vi "2_VisualAD__Inference(Image).vi"() -> ()   [LabVIEW 2020]
uses:
  <vilib>/Ngene/DeepLTK Anomaly Detection Addon/DeepLTK_Anomaly_Detection_Addon/API/Controls/NNPC_Setup.ctl
  <vilib>/Ngene/Deep Learning Toolkit/Toolkit/NN_Data/API/NN_Dims(C,H,W).ctl
  <vilib>/Ngene/Deep Learning Toolkit/Toolkit/NN_Network/Controls/NN_Device.ctl
  <vilib>/Ngene/DeepLTK Anomaly Detection Addon/DeepLTK_Anomaly_Detection_Addon/API/Controls/Feature_Scorer_Params.ctl
  <vilib>/Ngene/DeepLTK Anomaly Detection Addon/DeepLTK_Anomaly_Detection_Addon/API/Controls/Gaussian_Blur.ctl
  <vilib>/Ngene/DeepLTK Anomaly Detection Addon/DeepLTK_Anomaly_Detection_Addon/API/Controls/NN_Paths.ctl
  subVIs/Visualizer/Controls/Display_Options.ctl
  subVIs/Visualizer/Controls/ROI_Display_Options.ctl
  subVIs/Visualizer/Controls/Heatmap_Display_Options.ctl
  subVIs/Visualizer/Controls/ColorMap.ctl
  <vilib>/Ngene/DeepLTK Anomaly Detection Addon/DeepLTK_Anomaly_Detection_Addon/API/Controls/MinMax.ctl
  <vilib>/Ngene/DeepLTK Anomaly Detection Addon/DeepLTK_Anomaly_Detection_Addon/API/NNPC_Predict/NNPC_Predict(Single).vi
  <vilib>/ptbypt/NI_PtbyPt.lvlib
  <vilib>/Ngene/DeepLTK Anomaly Detection Addon/DeepLTK_Anomaly_Detection_Addon/DeepLTK_Anomaly_Detection_Addon.lvlib
  <vilib>/Ngene/Deep Learning Toolkit/Toolkit/Deep_Learning_Toolkit_by_Ngene.lvlib
panel:
  in  "Display_Options":T1={"ROI_Options"={"Color"=16383, "Width"=3, "Drawing Mode"=enum."Frame"}, "Heatmap_Options"={"ColorMap"=enum."Jet", "Alpha"=0.4, "Heatmap_Range"={"Min"=-1.0, "Max"=-1.0}}, "Has GT?"=FALSE} {"Heatmap_Options"."Heatmap_Range"."Min" format="%#_5g"}
  out "dT_Init":dbl=3.8699048000016774 format="%#_3ps"
  in  "NNPC_Paths":T6={"CFG"=path "D:/Ngene/GitHub/deepltk_examples/3_Image_Processing/36_Anomaly_Detection/Models/NNPC_Cards_3ofHearts__25_03_28__20_34_36/NNPC_Cards_3ofHearts.cfg", "BIN"=path "D:/Ngene/GitHub/deepltk_examples/3_Image_Processing/36_Anomaly_Detection/Models/NNPC_Cards_3ofHearts__25_03_28__20_34_36/NNPC_Cards_3ofHearts.bin"}
  out "Image_Thrshld (Eval)":sgl=11.161
  in  "Image_Thrshld(Custom)":sgl=-1.0 format="%_5g"
  out "dT_Predict":dbl=0.005395784000138519 format="%#_3ps"
  out "Pixel_Score(Min)":sgl=1.6810824
  out "Pixel_Score(Max)":sgl=12.34793
  out "Image_File_Path":path=path "D:/Ngene/GitHub/deepltk_examples/3_Image_Processing/36_Anomaly_Detection/Dataset/Playing_Cards_3ofHearts/test/bad/(159).png"
  in  "Feature_Scorer_Params":T7={"Nearest_Neighbors"=1, "Calculate Anomaly Map"=TRUE, "Gaussian_Blur"={"Kernel_Size"=33, "Sigma"=4.0}}
  out "Pixel_Thrshld (Eval)":sgl=2.5442
  in  "Stop":bool
  out "Anomaly?":bool=TRUE
  out "dT_ImRead":dbl=0.002829499997460516 format="%#_4ps"
  in  "NNPC_Setup":T9={"Input_Dims"={"C"=-1, "H"=-1, "W"=-1}, "mBatch"=1, "Device"=enum."GPU", "GPU Id"=0}
  out "Anomaly Detection Results":T12(plugin-control)
  out "Img_Score":sgl=14.09682
  in  "Image_idx":u32=33 max=49
  in  "Ground_Truth_Folder_Path":path
  in  "Pixel_Thrshld(Custom)":sgl=10.0 format="%_5g"
  in  "Test_Dataset_Folder_Path":path=path "D:/Ngene/GitHub/deepltk_examples/3_Image_Processing/36_Anomaly_Detection/Dataset/Playing_Cards_3ofHearts/test"
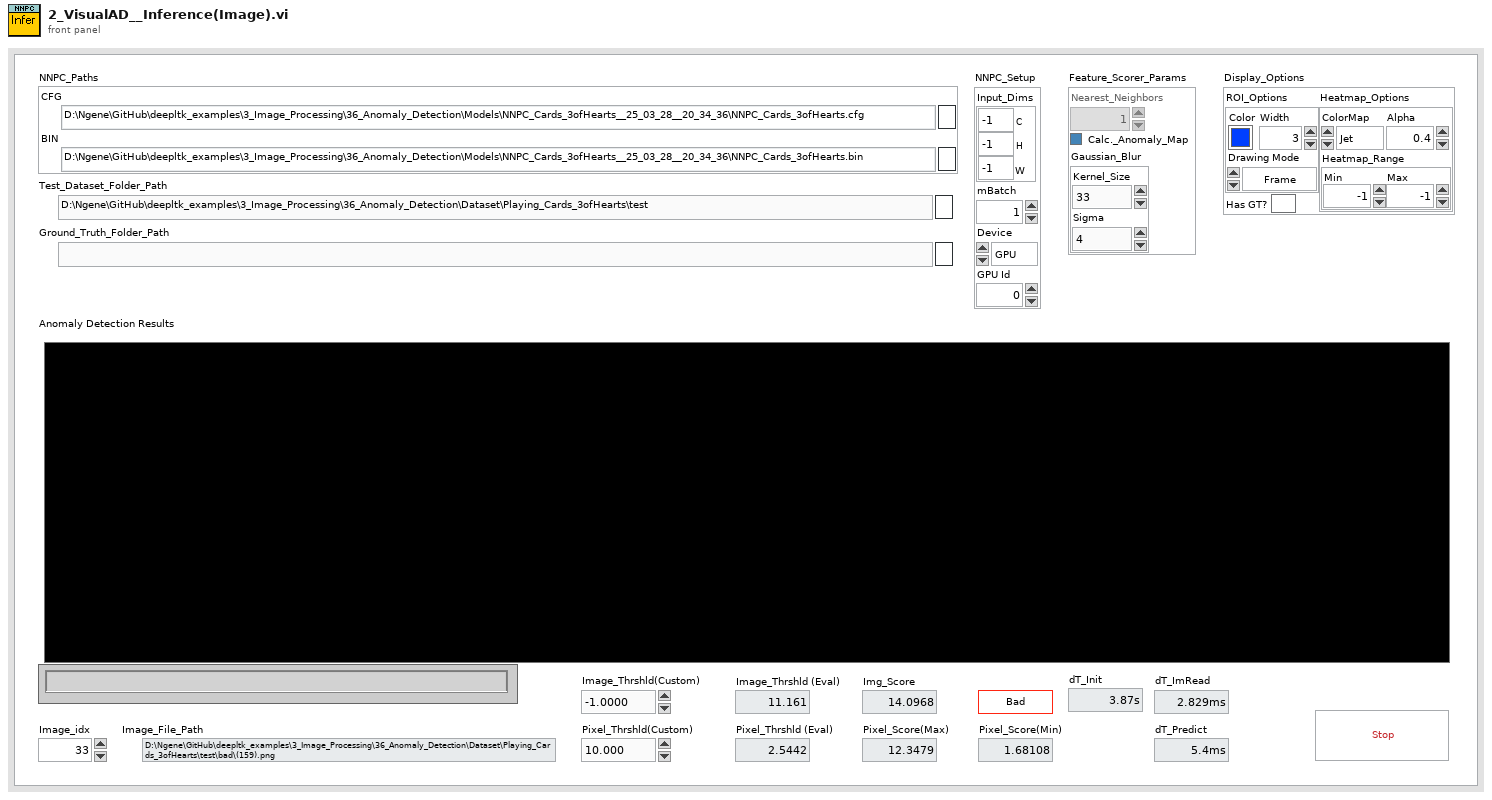
[diagram p1: front panel]
types:
  T1 = typedef "Display_Options.ctl" = cluster{"ROI_Options":T2, "Heatmap_Options":T3, "Has GT?":bool}
  T2 = typedef "ROI_Display_Options.ctl" = cluster{"Color":u32, "Width":u32, "Drawing Mode":enum16{"Frame", "Fill"}}
  T3 = typedef "Heatmap_Display_Options.ctl" = cluster{"ColorMap":T4, "Alpha":sgl, "Heatmap_Range":T5}
  T4 = typedef "ColorMap.ctl" = enum16{"Jet", "Perula", "Inferno", "Plasma", "Viridis"}
  T5 = typedef "DeepLTK_Anomaly_Detection_Addon.lvlib/MinMax.ctl" = cluster{"Min":sgl, "Max":sgl}
  T6 = typedef "DeepLTK_Anomaly_Detection_Addon.lvlib/NN_Paths.ctl" = cluster{"CFG":path, "BIN":path}
  T7 = typedef "DeepLTK_Anomaly_Detection_Addon.lvlib/Feature_Scorer_Params.ctl" = cluster{"Nearest_Neighbors":i32, "Calculate Anomaly Map":bool, "Gaussian_Blur":T8}
  T8 = typedef "DeepLTK_Anomaly_Detection_Addon.lvlib/Gaussian_Blur.ctl" = cluster{"Kernel_Size":i32, "Sigma":sgl}
  T9 = typedef "DeepLTK_Anomaly_Detection_Addon.lvlib/NNPC_Setup.ctl" = cluster{"Input_Dims":T10, "mBatch":i32, "Device":T11, "GPU Id":i32}
  T10 = typedef "Deep_Learning_Toolkit_by_Ngene.lvlib/NN_Dims(C,H,W).ctl" = cluster{"C":i32, "H":i32, "W":i32}
  T11 = typedef "Deep_Learning_Toolkit_by_Ngene.lvlib/NN_Device.ctl" = enum16{"CPU", "GPU"}
  T12 = typedef "IMAQ Image.ctl" = refnum<image>
  T13 = typedef "DeepLTK_Anomaly_Detection_Addon.lvlib/NNPC_Evaluation_Results.ctl" = cluster{"Threshold(Image)":sgl, "Threshold(Pixel)":sgl, "Pixel_Range":cluster{"Min":sgl, "Max":sgl}}
  T14 = typedef "DeepLTK_Anomaly_Detection_Addon.lvlib/NNPC_PreProcessing_Options.ctl" = cluster{"DS_Name":string, "Input_Dims":T10, "Center Crop Size":i32, "Interpolation Type":u32, "Dataset_Stats":T15}
  T15 = typedef "DeepLTK_Anomaly_Detection_Addon.lvlib/NNPC_DS_Stats.ctl" = cluster{"means":T16, "stds":T16}
  T16 = typedef "DeepLTK_Anomaly_Detection_Addon.lvlib/Image_Stats_RGB.ctl" = cluster{"R":sgl, "G":sgl, "B":sgl}
  T17 = typedef "DeepLTK_Anomaly_Detection_Addon.lvlib/NNPC_Instance.ctl" = cluster{"NN":T18, "MemBank_Data":T33, "Name":string}
  T18 = typedef "Deep_Learning_Toolkit_by_Ngene.lvlib/NN.ctl" = cluster{"Name":string, "No of Layers":i32, "mBatch":i32, "Layers":T19[], "Dimty":T20, "Dims_In":T10, "Dims_Out":T10, "Working_Dir":path, "Train?":bool, "Train_Params":T21, "LR_Update_Policy":T24, "Session Data":T26, "Ground_truth":T27, "NNg_hdls":T28, "NN_Device":T11, "GPU Id":i32, "Labels":string[], "Receptive Field":T29[], "Loss_Type":T30, "Loss_Cfg_Prms":variant, "NNG_WS":T31}
  T19 = typedef "Deep_Learning_Toolkit_by_Ngene.lvlib/NN_Layer_ref.ctl" = refnum<data-value>
  T20 = typedef "Deep_Learning_Toolkit_by_Ngene.lvlib/NN_In_Out_Dim-ty.ctl" = enum8{"In1D_Out1D", "In3D_Out1D", "In3D_Out3D", "In3D_OutBBox"}
  T21 = typedef "Deep_Learning_Toolkit_by_Ngene.lvlib/NN_Train_Params.ctl" = cluster{"Optimizer":T22, "Beta_1":sgl, "Beta_2":sgl, "Weight Decay(L1)":sgl, "Weight Decay(L2)":sgl, "Data_Sampling":T23}
  T22 = typedef "Deep_Learning_Toolkit_by_Ngene.lvlib/NN_Train_Optimizer.ctl" = enum16{"SGD", "Adam", "Adagrad", "Adadelta", "RMSProp", "Nesterov"}
  T23 = typedef "Deep_Learning_Toolkit_by_Ngene.lvlib/NN_Train_Data_Sampling.ctl" = enum16{"Random", "Sequential"}
  T24 = typedef "Deep_Learning_Toolkit_by_Ngene.lvlib/NN_LR_Policy_Cfg.ctl" = cluster{"Policy_Type":T25, "LR0":dbl, "k":sgl, "WarmUp_Policy":enum16{"Step", "Ramp"}, "WarmUp_Iter":i32, "WarmUp_Ratio":sgl}
  T25 = typedef "Deep_Learning_Toolkit_by_Ngene.lvlib/NN_LR_Policy_Type.ctl" = enum16{"Manual", "Step", "Exp", "1/t"}
  T26 = typedef "Deep_Learning_Toolkit_by_Ngene.lvlib/NN_Train_Session_Data.ctl" = cluster{"Epochs":sgl, "Tot_Iter":i32, "LR":sgl, "LR_iter":i32}
  T27 = typedef "Deep_Learning_Toolkit_by_Ngene.lvlib/NN_Ground_truth.ctl" = cluster{"Y":variant}
  T28 = typedef "Deep_Learning_Toolkit_by_Ngene.lvlib/nng_cuda_handles.ctl" = cluster{"cudnn":u64, "cublas":u64, "stream":u64, "curand":u64}
  T29 = typedef "Deep_Learning_Toolkit_by_Ngene.lvlib/NN_Dims(V,H).ctl" = cluster{"V":i32, "H":i32}
  T30 = typedef "Deep_Learning_Toolkit_by_Ngene.lvlib/NN_Loss_Type.ctl" = enum16{"None", "MSE", "CrossEntropy", "YOLO_v2", "YOLO_v4"}
  T31 = typedef "Deep_Learning_Toolkit_by_Ngene.lvlib/NNG_WS.ctl" = cluster{"NNG_WS_Mem":T32, "Max_WS_Size":i64}
  T32 = typedef "Deep_Learning_Toolkit_by_Ngene.lvlib/NNg_WS_Mem_DVR.ctl" = refnum<data-value>
  T33 = typedef "DeepLTK_Anomaly_Detection_Addon.lvlib/MemBank_and_Norm_Variants.ctl" = cluster{"MemBank":variant, "MemBank Norm":variant}
  T34 = typedef "Anomaly_Detection_Results_Imgs.ctl" = cluster{"Image":T12, "Ground Truth":T12, "Predicted Heat Map":T12, "Predicted Mask":T12, "Segmentation":T12}
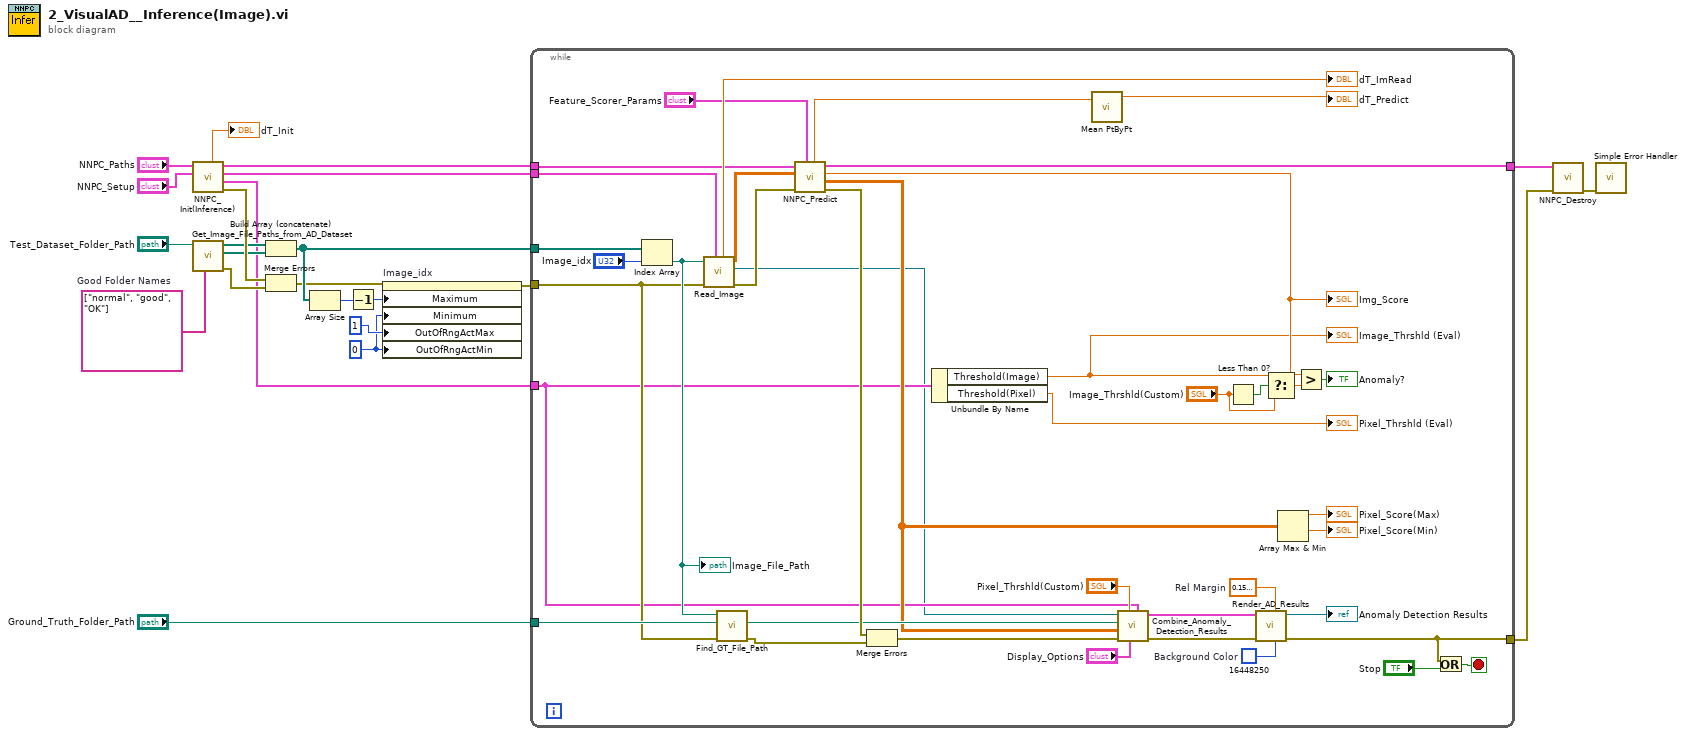
[diagram p0: block diagram]
diagram:
  w1 = string[] ["normal", "good", "OK"]  # Good Folder Names
  w3 = u32 0 ("Data Entry Limits:Minimum")
  n1 = call <vilib>:"NNPC_Init(Inference).vi"("NNPC_Setup"="NNPC_Setup", "NNPC_Paths"="NNPC_Paths") -> ("error out"=w21:errorcluster, "Evaluation_Results"=w4:T13, "PreProc_Options"=w6:T14, "NNPC_out"=w22:T17, "dT_Init_Inference"=→"dT_Init":dbl)  [unwired: 5 in]
  n2 = call "Get_Image_File_Paths_from_AD_Dataset.vi"("Good Folder Names"=w1, "Dataset Folder"="Test_Dataset_Folder_Path") -> ("error out"=w18:errorcluster, "Bad Dataset Files"=w14:path[], "Good Dataset Files"=w13:path[])  [unwired: 7 in]
  n3 = Build Array (concatenate)(w13, w14) -> (w19:path[])
  n4 = Merge Errors(w21, w18) -> (w8:errorcluster)
  n5 = Array Size(array=w19) -> (size(s)=w9:i32)
  n6 = Decrement(x=w9) -> (x-1=w11:i32)
  n7 = property on="Image_idx" class="DigNum (strict)"(error in=w8, "Maximum"=w11, "Minimum"=w3, "OutOfRngActMax"=u8 1 ("Response to Value Outside Limits:Maximum"), "OutOfRngActMin"=w3) -> (error out=w7:errorcluster)  [unwired: 1 in, 1 out]
  n8 = while {
    tunnel: w19 -> [w63]
    tunnel: w22 -> [w45]
    tunnel: [w39] -> w16
    tunnel: w7 -> [w34]
    tunnel: [w36] -> w17
    tunnel: "Ground_Truth_Folder_Path" -> [w48]
    tunnel: w6 -> [w31]
    tunnel: w4 -> [w27]
    stop <- w37 stop-if-true
    w35 = u32 16448250  # Background Color
    w55 = sgl 0.15  # Rel Margin
    n9 = Index Array(array=w63, index="Image_idx") -> (element=w50:path)
    "Image_File_Path" <- w50
    n10 = call "Read_Image.vi"("PreProcessing_Options"=w31, "error in"=w34, "Img Path"=w50) -> ("error out"=w40:errorcluster, "Imaq Image Out"=w26:T12, "Image Out"=w24:sgl[][][], "dT_Img_Read"=→"dT_ImRead":dbl)  [unwired: 5 in]
    n11 = call "Find_GT_File_Path.vi"("error in"=w34, "GT Mask Folder Path"=w48, "Image File Path"=w50) -> ("error out"=w32:errorcluster, "GT File Path"=w49:path)  [unwired: 5 in, 2 out]
    n12 = call-poly <vilib>:"NNPC_Predict.vi"("Feature_Scorer_Params"="Feature_Scorer_Params", "error in"=w40, "Image_in"=w24, "NNPC_in"=w45) -> ("error out"=w61:errorcluster, "Anomaly_Map"=w44:sgl[][], "Pred_Score"=w43:sgl, "NNPC_out"=w39:T17, "dT_Predict"=w30:dbl)  [unwired: 3 in]
    "Img_Score" <- w43
    n13 = Merge Errors(w61, w32) -> (w33:errorcluster)
    n14 = Unbundle By Name(w27) -> ("Threshold(Image)"=w29:sgl, "Threshold(Pixel)"=→"Pixel_Thrshld (Eval)":sgl)
    "Image_Thrshld (Eval)" <- w29
    n15 = call <vilib>:"Mean PtByPt.vi"("x"=w30) -> ("mean"=→"dT_Predict":dbl)  [unwired: 3 in, 1 out]
    n16 = call "Combine_Anomaly_Detection_Results.vi"("Evaluation_Results"=w27, "Display_Options"="Display_Options", "Pixel Anomaly Thrshld"="Pixel_Thrshld(Custom)", "error in"=w33, "Anomaly Map"=w44, "Gt File Path"=w49, "Orig Image In"=w26) -> ("error out"=w60:errorcluster, "Anomaly Detection Rresults"=w59:T34)  [unwired: 2 in, 1 out]
    n17 = Less Than 0?(x="Image_Thrshld(Custom)") -> (x < 0?=w54:bool)
    n18 = call "Render_AD_Results.vi"("Background Color"=w35, "Rel._Margin"=w55, "error in"=w60, "Anomaly Detection Rresults"=w59) -> ("error out"=w36:errorcluster, "Anomaly Detection Results"=→"Anomaly Detection Results":T12)  [unwired: 6 in]
    n19 = Select(t=w29, s=w54, f="Image_Thrshld(Custom)") -> (s? t:f=w52:sgl)
    n20 = Array Max & Min(array=w44) -> (max value=→"Pixel_Score(Max)":sgl, min value=→"Pixel_Score(Min)":sgl)  [unwired: 2 out]
    n21 = Greater?(x=w43, y=w52) -> (0:→"Anomaly?":bool)
    n22 = Or(x=w36, y="Stop") -> (x .or. y?=w37:bool)
  }
  n23 = call <vilib>:"NNPC_Destroy.vi"("error in"=w17, "NNPC_in"=w16) -> ("error out"=w15:errorcluster)  [unwired: 9 in]
  n24 = call <vilib>:"Simple Error Handler.vi"("error in (no error)"=w15) -> ()  [unwired: 4 in, 5 out]
